vi "2100_Test_Guardian Switch_No Publish Data.vi"(0 "Semiconductor Module Context":T6, 1 "Current  Level":dbl=0.01, 2 "Master_Register_Data_Array_In":T1 {"Address" format="%.0x"}, 5 "Script_Info":T4={"Script Name"="WalkingState", "All_Scripts"=[]}, 9 "USID":T3 max=15, 11 "Error In":errorcluster, 12 "Instrument_Pins":T5={"SMU_Pins"=["RF1", "RF2", "RF3", "RF4"], "HSDIO_Pins"=["CLK", "SDA"]}, 13 "Reg_Map_Bit_Name":string="RFC_SH", 14 "Reg_Map":string[][](array[string])=[["Reg Addr(0x00)", "7", "6", "5", "4", "3", "2", "1", "0"], ["0", "SPARE", "RF3_SH", "RF2_SH", "RF1_SH", "SPARE", "RF3_RFC", "RF2_RFC", "RF1_RFC"], ["1", "SPARE[7:0]", "", "", "", "", "", "", ""], ["2", "VVAR_EN", "LCM_EN", "RFC_SH", "SPARE", "VARACTOR[3:0]", "", "", ""], ["3", "SW_CTRL1_VIRTUAL[7:0]", "", "", "", "", "", "", ""], ["4", "SW_CTRL1_SWAP", "SW_CTRL1_RBSHIFT[2:0]", "", "", "SW_CTRL1_VSID[3:0]", "", "", ""], ["5", "REG_00_VIRTUAL_MASK[7:0]", "", "", "", "", "", "", ""], ["6", "LOCK_STATUS[1:0]", "", "CLK_DITHER", "FUSES_BURNED", "CLK_IDAC_CAL[3:0]", "", "", ""], ["7", "SPARE[2:0]", "", "", "ODFT_TRIM[4:0]", "", "", "", ""], ["8", "SPARE[2:0]", "", "", "HV_TRIM[4:0]", "", "", "", ""], ["9", "TEST_MUX[2:0]", "", "", "SPARE[1:0]", "", "MEMS_BG_TC[1:0]", "", "MEMSCP_RCM"], ["A", "CP_BOOST_OVRD_EN", "SPARE[2:0]", "", "", "PS_OFF_TIMER[1:0]", "", "PS_ON_TIMER[1:0]", ""], ["0", "", "", "", "", "", "", "", ""], ["D", "Reserved[1:0]", "", "WD_HI_EVENT_CNT[5:0]", "", "", "", "", ""], ["E", "VERSION_ID[7:0]", "", "", "", "", "", "", ""], ["F", "Reserved", "COUNT_200_LSB[6:0]", "", "", "", "", "", ""], ["10", "CLK_DIV2_EN", "Spare", "ODFT_EN", "HV_HYST[4:0]", "", "", "", ""], ["0", "", "", "", "", "", "", "", ""], ["12", "SHORT_FUSE", "FUSE_BURN", "STROBE_EN", "VIO_OK", "RTH[1:0]", "", "FUSE_LOAD_MAN_EN", "FUSE_LOAD"], ["13", "RR_ACK_EN", "Reserved", "ACK_POSITION[1:0]", "", "SuBUS_DRIVE_STRENGTH[3:0]", "", "", ""], ["14", "TM_IO_EN", "TM_IO_SEL", "SuBUS_OVS[1:0]", "", "Reserved[3:0]", "", "", ""], ["15", "Reserved[4:0]", "", "", "", "", "SuBUS_VERSION_PRESENT", "SuBUS_VOLTAGE", "SuBUS_FLAVOR_DEF"], ["16", "PROG_STROBE1_DUR[7:0]", "", "", "", "", "", "", ""], ["17", "PROG_STROBE0_DUR[7:0]", "", "", "", "", "", "", ""], ["18", "Reserved[2:0]", "", "", "EFUSE_SINGLE_ADDR_SEL[4:0]", "", "", "", ""], ["19", "POLL_ADR[4:0]", "", "", "", "", "POLL_BC[2:0]", "", ""], ["1A", "SOFTWARE_RESET", "Reserved[6:0]", "", "", "", "", "", ""], ["1B", "Reserved[7:0]", "", "", "", "", "", "", ""], ["1C", "PWR_MODE_1", "PWR_MODE_0", "TRIGGER_MASK[2:0]", "", "", "TRIGGER[2:0]", "", ""], ["1D", "PRODUCT_ID[7:0]", "", "", "", "", "", "", ""], ["1E", "MANUFACTURER_ID_LSB[7:0]", "", "", "", "", "", "", ""], ["1F", "MANUFACTURER_ID_MSB[3:0]", "", "", "", "USID[3:0]", "", "", ""]]) -> (6 "Master_Register_Data_Array_Out":T1 {"Address" format="%.0x"}, 8 "R_Guardian":dbl[](array[numeric]), 15 "Error Out":errorcluster)   [LabVIEW 2013]
uses:
  Controls/USID.ctl
  <vilib>/NI_TestStand_SemiconductorModule/NI_TestStand_Semiconductor_Module.lvlibp/PinMap/General/SemiconductorModuleContext.ctl
  Controls/Master_Reg_Data_Array.ctl
  Controls/Reg_Address_Data.ctl
  <vilib>/NI_TestStand_SemiconductorModule/NI_TestStand_Semiconductor_Module.lvlibp
panel:
  out "R Array":dbl[][](array[numeric])
  in  "Tab Control":enum32{"Test Info", "Instrument Settings"}(tab)
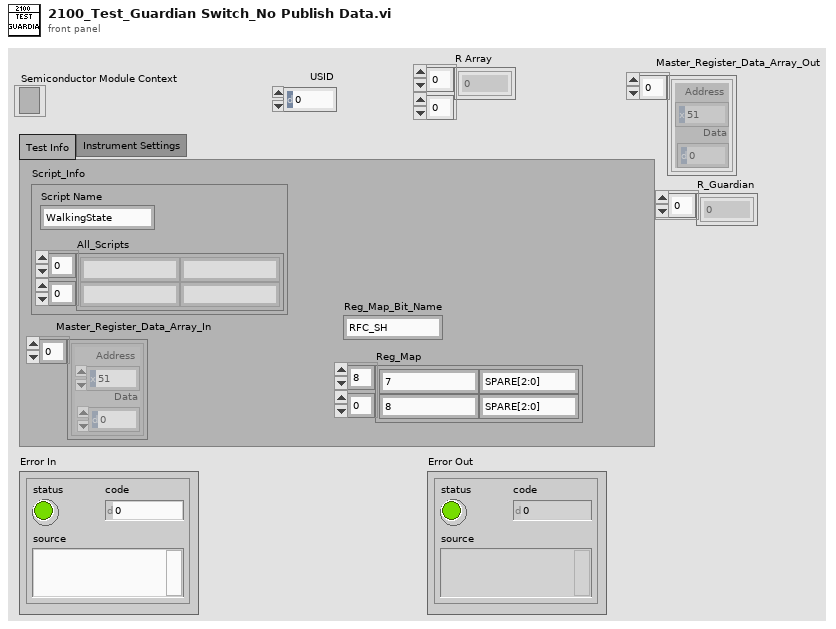
[diagram p1: front panel]
types:
  T1 = typedef "Master_Reg_Data_Array.ctl" = T2[]
  T2 = typedef "Reg_Address_Data.ctl" = cluster{"Address":u8, "Data":u8}
  T3 = typedef "USID.ctl" = u8
  T4 = cluster{"Script Name":string, "All_Scripts":string[][]}
  T5 = cluster{"SMU_Pins":string[], "HSDIO_Pins":string[]}
  T6 = typedef "NI_TestStand_Semiconductor_Module.lvlibp/SemiconductorModuleContext.ctl" = refnum<k7>
  T7 = typedef "Script Functions_Array.ctl" = enum16{"Reg_Write", "Bit_Write", "Delay", "Read", "Measure"}[]
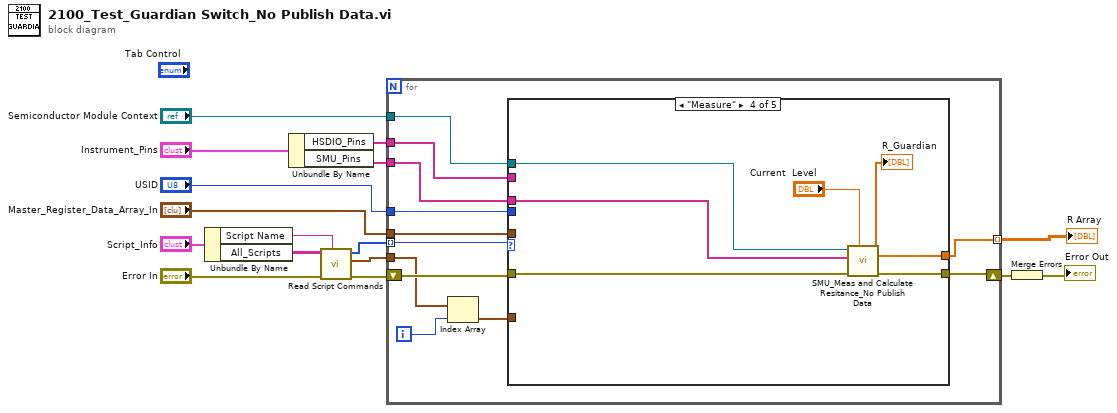
[diagram p0: block diagram]
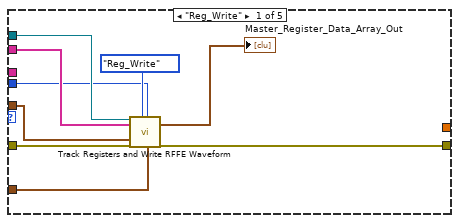
[diagram p2: hidden frame]
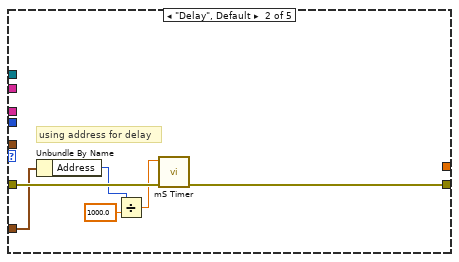
[diagram p3: hidden frame]
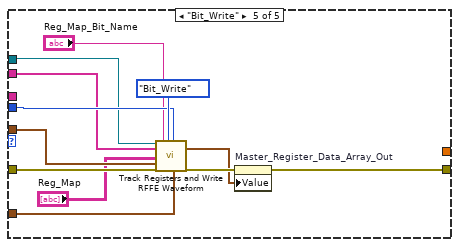
[diagram p5: hidden frame]
diagram:
  n1 = Unbundle By Name("Script_Info") -> ("Script Name"=w1:string, "All_Scripts"=w2:string[][])
  n2 = Unbundle By Name("Instrument_Pins") -> ("HSDIO_Pins"=w5:string[], "SMU_Pins"=w4:string[])
  n3 = call "Read Script Commands.vi"("Test Name"=w1, "Error In"="Error In", "All_Scripts"=w2) -> ("Error Out"=w13:errorcluster, "Script_Data"=w14:T2[], "Script_Functions"=w15:T7)  [unwired: 5 in, 1 out]
  n4 = for {
    tunnel: "USID" -> [w22]
    tunnel: w15 -> [w21] mode=indexing
    tunnel: w14 -> [w25]
    tunnel: "Semiconductor Module Context" -> [w27]
    tunnel: w5 -> [w26]
    shift-right: [w18] -> w9
    shift-left: w13 -> [w28]
    tunnel: "Master_Register_Data_Array_In" -> [w23]
    tunnel: w4 -> [w17]
    tunnel: [w19] -> w10 mode=indexing
    i -> [w20]
    n5 = Index Array(array=w25, index=w20) -> (element=w24:T2)
    n6 = case shown="\"Measure\"" w21 {
      tunnel: w24 -> [w32 w42 _ _ w55]
      tunnel: w28 -> [w37 w43 w44 w50 w62]
      tunnel: w22 -> [w29 _ _ _ w60]
      tunnel: w27 -> [w35 _ _ w46 w59]
      tunnel: w26 -> [w34 _ _ _ w58]
      tunnel: [w36 w41 w44 w49 w52] -> w18
      tunnel: w23 -> [w31 _ _ _ w56]
      tunnel: [_ _ _ w47 _] -> w19
      tunnel: w17 -> [_ _ _ w45 _]
      frame "Reg_Write" {
        n7 = call "Track Registers and Write RFFE Waveform.vi"("Semiconductor Module Context"=w35, "Pins"=w34, "Master_Register_Data_Array_In"=w31, "Error In"=w37, "Script_Functions"=enum16{"Reg_Write", "Bit_Write"}."Reg_Write", "USID"=w29, "Reg_Address_Data"=w32) -> ("Master_Register_Data_Array_Out"=→"Master_Register_Data_Array_Out":T1, "Error Out"=w36:errorcluster)  [unwired: 10 in, 1 out]
      }
      frame "Delay", Default {
        # "using address for delay"
        n8 = Unbundle By Name(w42) -> ("Address"=w39:u8)
        n9 = Divide(x=w39, y=1000.0) -> (x/y=w38:dbl)
        n10 = call "mS Timer.vi"("Error In"=w43, "Delay(S)"=w38) -> ("Error Out"=w41:errorcluster)  [unwired: 9 in]
      }
      frame "Read" {
      }
      frame "Measure" {
        n11 = call "SMU_Meas and Calculate Resitance_No Publish Data.vi"("Current  Level"="Current  Level", "error in (no error)"=w50, "Pins"=w45, "Semiconductor Module Context"=w46) -> ("error Out"=w49:errorcluster, "R Array"=w47:dbl[])  [unwired: 5 in, 1 out]
        "R_Guardian" <- w47
      }
      frame "Bit_Write" {
        n12 = call "Track Registers and Write RFFE Waveform.vi"("Semiconductor Module Context"=w59, "Pins"=w58, "Reg_Map"="Reg_Map", "Master_Register_Data_Array_In"=w56, "Error In"=w62, "Reg_Map_Bit_Name"="Reg_Map_Bit_Name", "Script_Functions"=enum16{"Reg_Write", "Bit_Write"}."Bit_Write", "USID"=w60, "Reg_Address_Data"=w55) -> ("Master_Register_Data_Array_Out"=w51:T1, "Error Out"=w53:errorcluster)  [unwired: 8 in, 1 out]
        n13 = property on="Master_Register_Data_Array_Out" class="Arr (strict)"(error in=w53, "Value"=w51) -> (error out=w52:errorcluster)  [unwired: 1 in, 1 out]
      }
    }
  }
  "R Array" <- w10
  n14 = Merge Errors(w9) -> (→"Error Out":errorcluster)
